vi "StahlPS_USB.ProcCases.vi"(0 "i ref in":refnum<vi>, 1 "selector":string, 2 "Data":T1, 3 "call cluster":T2={"Object"="", "Selector"="", "CallType"=enum."synchronous", "Async Object"="", "Async Selector"="", "Data Descriptor"="", "Data"=[], "Error #"=0, "Expire"=0}, 5 "error in (no error)":errorcluster) -> (14 "i ref out":refnum<vi>, 17 "answer cluster":T2={"Object"="", "Selector"="", "CallType"=enum."synchronous", "Async Object"="", "Async Selector"="", "Data Descriptor"="", "Data"=[], "Error #"=0, "Expire"=0}, 19 "error out":errorcluster)   [LabVIEW 2014, in "StahlPS_USB.lvlib"]
doc: "This method is called by a process from within the default case in the event loop. The methods of a class that are linked to events will be called from THIS method. Add your code here."
uses:
  StahlPS_USB.lvlib
  CSCore/CSSystem/CoreLib/CoreLib.lvlib
  CSCore/BaseProcess/BaseProcess.lvlib
  CSCore/CSSystem/CoreLib/CoreLib.byte array 2 double.vi
  CSCore/CSSystem/CoreLib/CoreLib.string 2 byte array.vi
  CSCore/CSApplicationBaseClasses/PSChannelBase/PSChannelBase.lvlib
  CSCore/CSSystem/CoreLib/CoreLib.byte array 2 int.vi
  CSCore/CSSystem/CoreDefs/CoreDefs.call_type.ctl
  CSCore/CSSystem/CoreDefs/CoreDefs.rawDataType.ctl
  CSCore/BaseProcess/BaseProcess.descriptor string definition.ctl
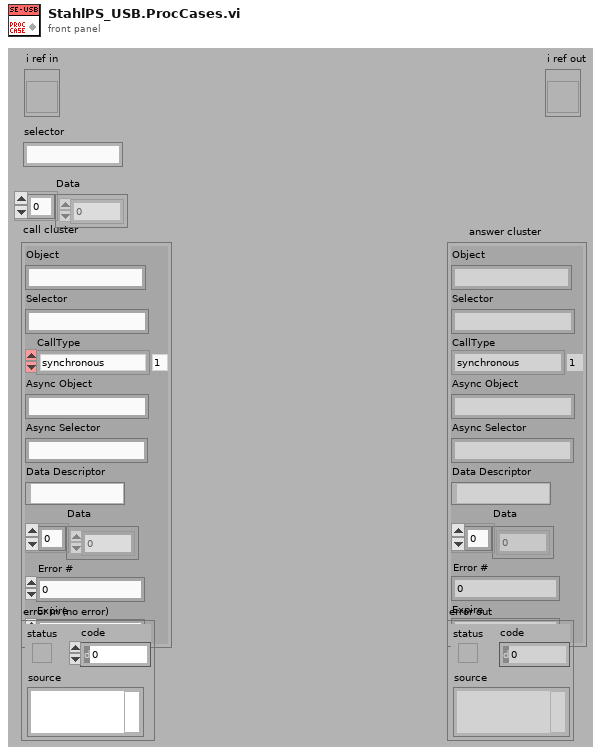
[diagram p1: front panel]
types:
  T1 = typedef "CoreDefs.rawDataType.ctl" = i8[]
  T2 = typedef "CoreDefs.call_type.ctl" = cluster{"Object":string, "Selector":string, "CallType":enum16{"simple", "synchronous", "asynchronous"}, "Async Object":string, "Async Selector":string, "Data Descriptor":T3, "Data":T1, "Error #":i32, "Expire":u32}
  T3 = typedef "BaseProcess.lvlib/BaseProcess.descriptor string definition.ctl" = string
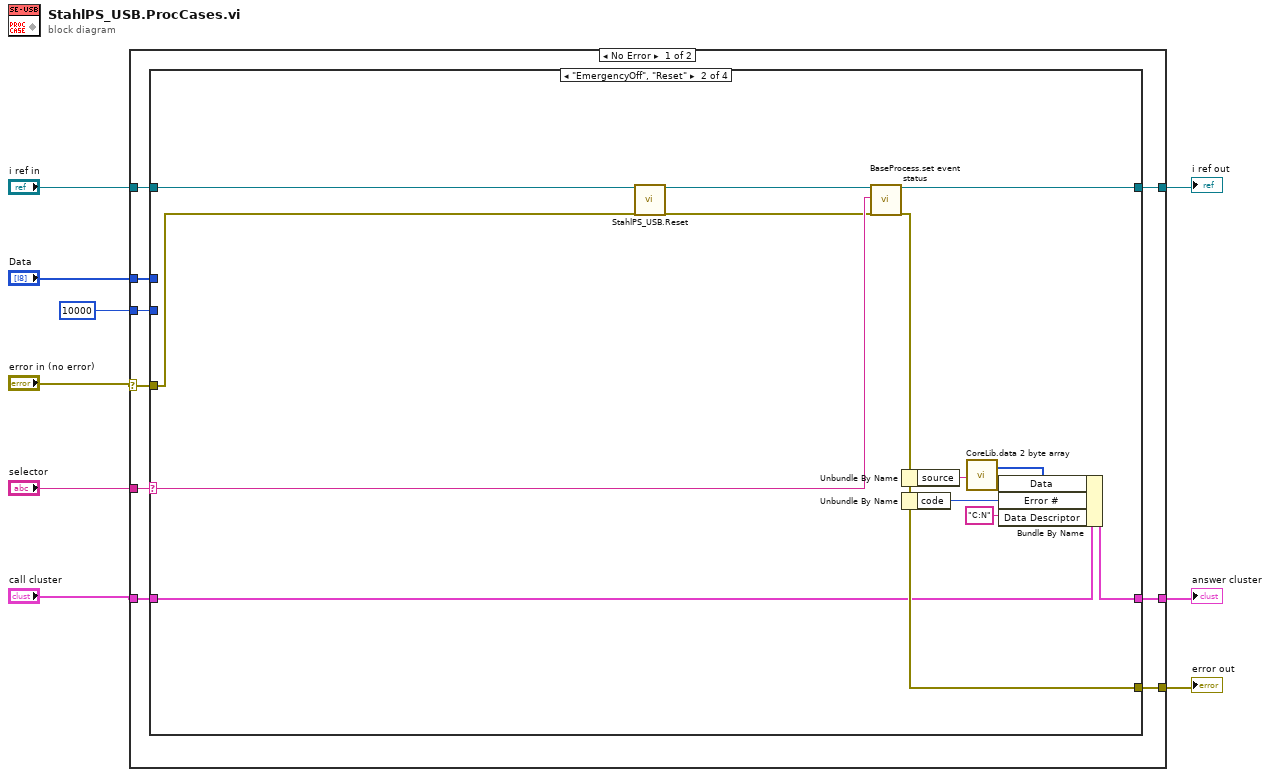
[diagram p0: block diagram]
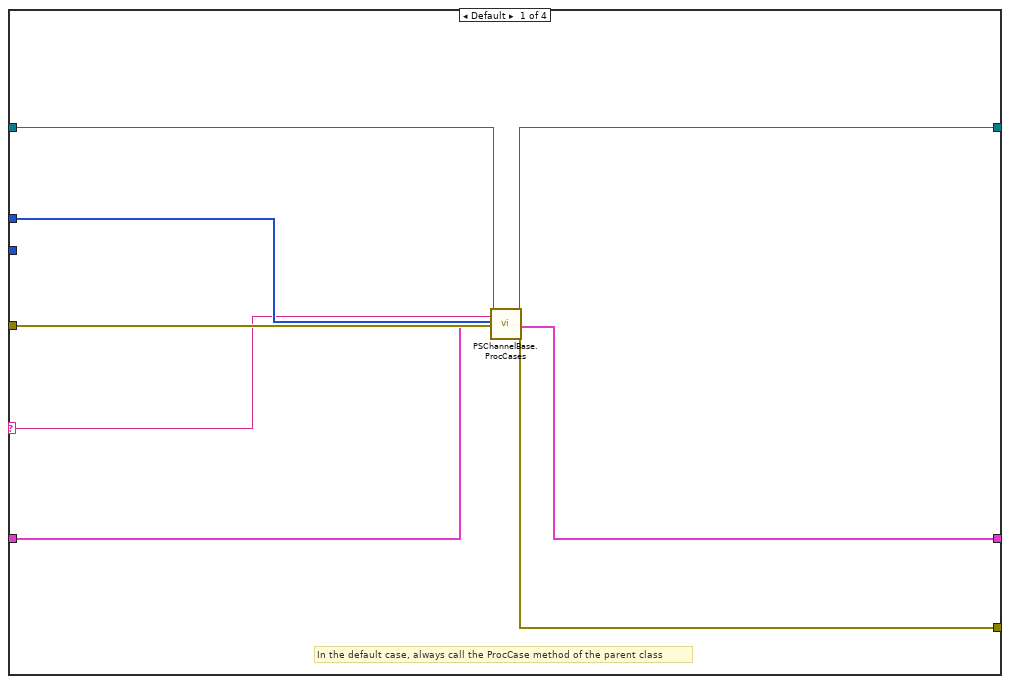
[diagram p2: hidden frame]
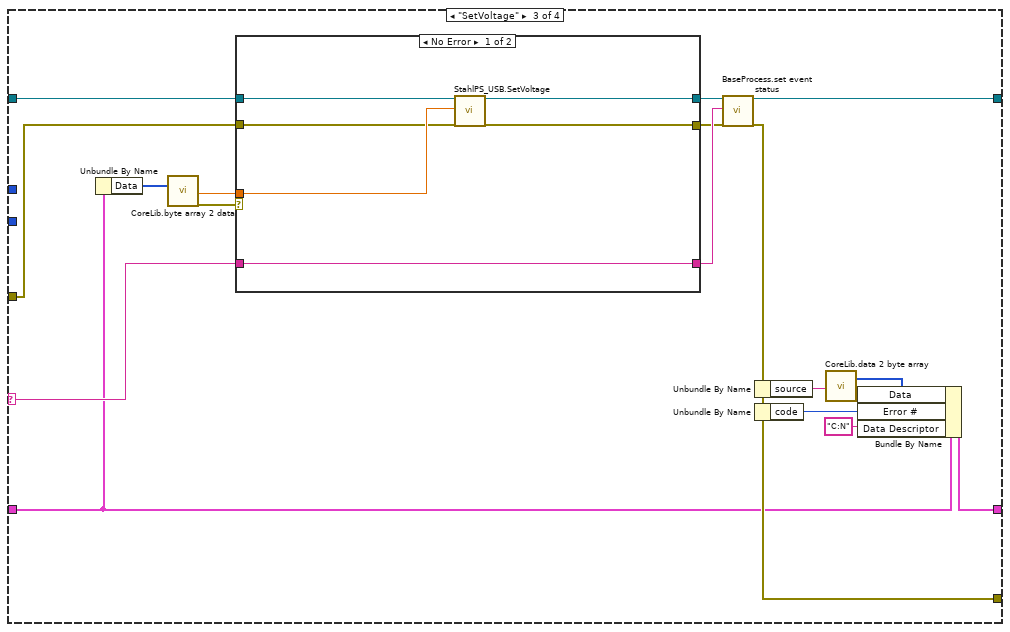
[diagram p3: hidden frame]
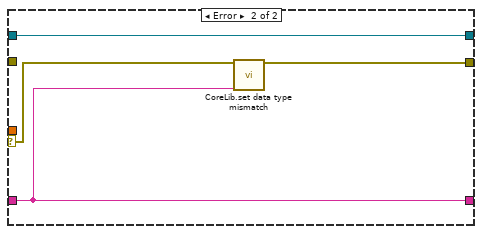
[diagram p4: hidden frame]
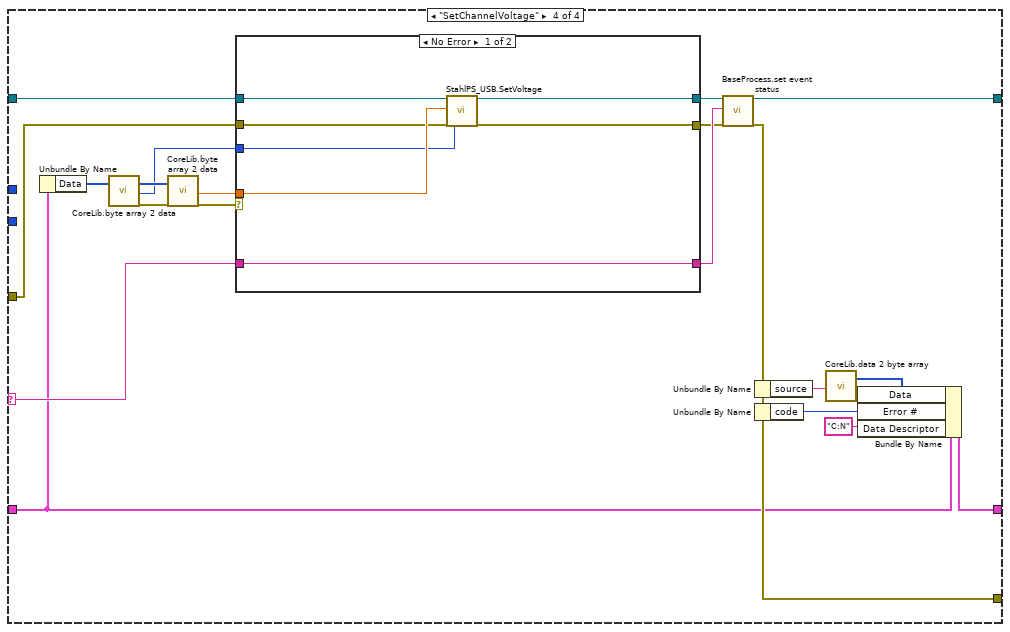
[diagram p5: hidden frame]
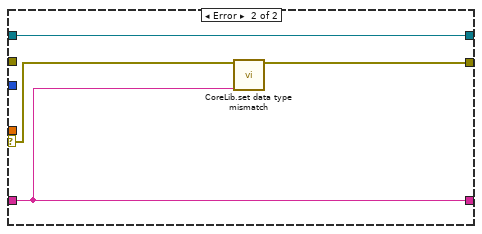
[diagram p6: hidden frame]
diagram:
  n1 = case shown="No Error" "error in (no error)" {
    selector: "error in (no error)" -> [w11 w98]
    tunnel: "selector" -> [w18 _]
    tunnel: [w17 w99] -> w3
    tunnel: "Data" -> [w16 _]
    tunnel: "call cluster" -> [w15 w99]
    tunnel: "i ref in" -> [w14 w100]
    tunnel: [w13 w100] -> w4
    tunnel: [w12 w98] -> w2
    tunnel: 10000 ("ms timeout (100)") -> [w10 _]
    frame No Error {
      n2 = case shown="\"EmergencyOff\", \"Reset\"" w18 {
        selector: w18 -> [w20 w36 w51 w81]
        tunnel: w16 -> [w21 _ _ _]
        tunnel: w14 -> [w19 w38 w55 w85]
        tunnel: [w26 w39 w56 w86] -> w13
        tunnel: w15 -> [w22 w28 w41 w72]
        tunnel: [w23 w30 w46 w76] -> w17
        tunnel: w11 -> [w25 w27 w40 w71]
        tunnel: [w24 w29 w45 w75] -> w12
        tunnel: w10 -> [_ _ _ _]
        frame Default {
          # "In the default case, always call the ProcCase method of the parent class"
          n3 = call "PSChannelBase.ProcCases.vi"("i ref in"=w19, "selector"=w20, "Data"=w21, "call cluster"=w22, "error in (no error)"=w25) -> ("i ref out"=w26:refnum<vi>, "answer cluster"=w23:T2, "error out"=w24:errorcluster)  [unwired: 12 in]
        }
        frame "EmergencyOff", "Reset" {
          n4 = call "StahlPS_USB.Reset.vi"("i ref in"=w38, "error in (no error)"=w27) -> ("i ref out"=w37:refnum<vi>, "error out (no error)"=w35:errorcluster)  [unwired: 16 in]
          n5 = call "BaseProcess.set event status.vi"("i ref in"=w37, "EventStatus"=w36, "error in (no error)"=w35) -> ("i ref out"=w39:refnum<vi>, "error out"=w29:errorcluster)  [unwired: 14 in, 1 out]
          n6 = Unbundle By Name(w29) -> ("source"=w31:string)
          n7 = Unbundle By Name(w29) -> ("code"=w34:i32)
          n8 = call-poly "CoreLib.data 2 byte array.vi"("string"=w31) -> ("byteArray out"=w33:T1)  [unwired: 18 in]
          n9 = Bundle By Name(cluster=w28, "Data"=w33, "Error #"=w34, "Data Descriptor"="C:N") -> (w30:T2)
        }
        frame "SetVoltage" {
          n10 = Unbundle By Name(w41) -> ("Data"=w44:T1)
          n11 = call-poly "CoreLib.byte array 2 data.vi"("byteArray"=w44) -> ("d64"=w42:dbl, "error out"=w43:errorcluster)  [unwired: 16 in, 1 out]
          n12 = case shown="No Error" w43 {
            selector: w43 -> [_ w66]
            tunnel: w51 -> [w59 w65]
            tunnel: [w59 w65] -> w53
            tunnel: [w60 w64] -> w52
            tunnel: w55 -> [w62 w63]
            tunnel: [w61 w63] -> w54
            tunnel: w42 -> [w58 _]
            tunnel: w40 -> [w57 _]
            frame No Error {
              n13 = call "StahlPS_USB.SetVoltage.vi"("i ref in"=w62, "value"=w58, "error in (no error)"=w57) -> ("i ref out"=w61:refnum<vi>, "error out (no error)"=w60:errorcluster)  [unwired: 15 in]
            }
            frame Error {
              n14 = call "CoreLib.set data type mismatch.vi"("error in (no error)"=w66, "error source"=w65) -> ("error out"=w64:errorcluster)  [unwired: 17 in]
            }
          }
          n15 = call "BaseProcess.set event status.vi"("i ref in"=w54, "EventStatus"=w53, "error in (no error)"=w52) -> ("i ref out"=w56:refnum<vi>, "error out"=w45:errorcluster)  [unwired: 14 in, 1 out]
          n16 = Unbundle By Name(w45) -> ("source"=w47:string)
          n17 = Unbundle By Name(w45) -> ("code"=w50:i32)
          n18 = call-poly "CoreLib.data 2 byte array.vi"("string"=w47) -> ("byteArray out"=w49:T1)  [unwired: 18 in]
          n19 = Bundle By Name(cluster=w41, "Data"=w49, "Error #"=w50, "Data Descriptor"="C:N") -> (w46:T2)
        }
        frame "SetChannelVoltage" {
          n20 = Unbundle By Name(w72) -> ("Data"=w70:T1)
          n21 = call-poly "CoreLib.byte array 2 data.vi"("byteArray"=w70) -> ("byteArray out"=w68:T1, "i32"=w67:i32, "error out"=w69:errorcluster)  [unwired: 16 in]
          n22 = call-poly "CoreLib.byte array 2 data.vi"("byteArray"=w68, "error in (no error)"=w69) -> ("d64"=w73:dbl, "error out"=w74:errorcluster)  [unwired: 15 in, 1 out]
          n23 = case shown="No Error" w74 {
            selector: w74 -> [_ w97]
            tunnel: w81 -> [w90 w96]
            tunnel: [w90 w96] -> w83
            tunnel: [w91 w95] -> w82
            tunnel: w85 -> [w93 w94]
            tunnel: [w92 w94] -> w84
            tunnel: w73 -> [w89 _]
            tunnel: w71 -> [w88 _]
            tunnel: w67 -> [w87 _]
            frame No Error {
              n24 = call "StahlPS_USB.SetVoltage.vi"("i ref in"=w93, "value"=w89, "error in (no error)"=w88, "channelIndex"=w87) -> ("i ref out"=w92:refnum<vi>, "error out (no error)"=w91:errorcluster)  [unwired: 14 in]
            }
            frame Error {
              n25 = call "CoreLib.set data type mismatch.vi"("error in (no error)"=w97, "error source"=w96) -> ("error out"=w95:errorcluster)  [unwired: 17 in]
            }
          }
          n26 = call "BaseProcess.set event status.vi"("i ref in"=w84, "EventStatus"=w83, "error in (no error)"=w82) -> ("i ref out"=w86:refnum<vi>, "error out"=w75:errorcluster)  [unwired: 14 in, 1 out]
          n27 = Unbundle By Name(w75) -> ("source"=w77:string)
          n28 = Unbundle By Name(w75) -> ("code"=w80:i32)
          n29 = call-poly "CoreLib.data 2 byte array.vi"("string"=w77) -> ("byteArray out"=w79:T1)  [unwired: 18 in]
          n30 = Bundle By Name(cluster=w72, "Data"=w79, "Error #"=w80, "Data Descriptor"="C:N") -> (w76:T2)
        }
      }
    }
    frame Error {
    }
  }
  "answer cluster" <- w3
  "i ref out" <- w4
  "error out" <- w2
